vi "TEST - Write INI Cluster.vi"(8 "error in (no error)":errorcluster) -> (0 "error out":errorcluster, 2 "Passed":bool)   [LabVIEW 2009]
uses:
  <vilib>/Utility/config.llb/NI_LVConfig.lvlib
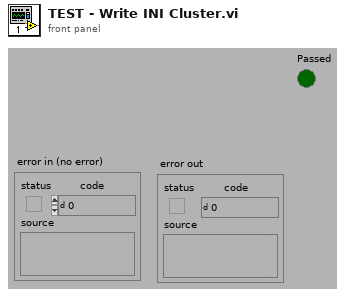
[diagram p1: front panel]
types:
  T1 = cluster{"Section 1":cluster{"Float":dbl, "Integer":i32}, "Section 2":cluster{"Boolean":bool, "String":string}}
  T2 = typedef "NI_LVConfig.lvlib/Config Data RefNum.ctl" = refnum<k1>
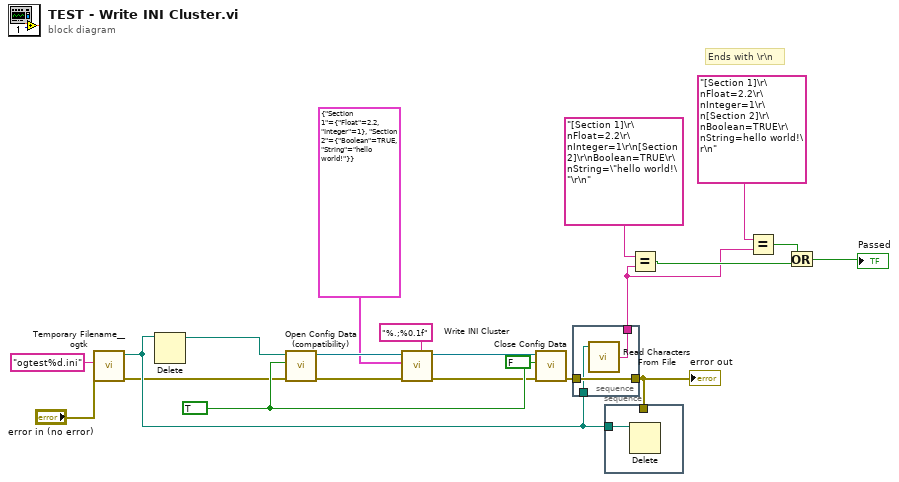
[diagram p0: block diagram]
diagram:
  (unwired) FALSE ("write configuration file? (T)")
  w19 = TRUE ("create file if necessary? (T)")
  # "Ends with \\r\\n"
  n1 = call <userlib>:"Temporary Filename__ogtk.vi"("error in (no error)"="error in (no error)", "pattern (lvtemp%d.tmp)"="ogtest%d.ini") -> ("error out"=w7:errorcluster, "file in tmp dir"=w8:path)  [unwired: 4 in]
  n2 = Delete(path (use dialog)=w8) -> (deleted path=w17:path)  [unwired: 4 in, 2 out]
  n3 = call <vilib>:"Open Config Data (compatibility).vi"("error in (no error)"=w7, "create file if necessary (T)"=w19, "configuration file path"=w17) -> ("error out"=w15:errorcluster, "refnum"=w16:T2)  [unwired: 6 in, 1 out]
  n4 = call "Write INI Cluster.vi"("float number format (optional)"="%.;%0.1f", "error in (no error)"=w15, "INI Fomatted Cluster"=T1 {"Section 1"={"Float"=2.2, "Integer"=1}, "Section 2"={"Boolean"=TRUE, "String"="hello world!"}}, "refnum"=w16) -> ("error out"=w18:errorcluster, "dup refnum"=w20:T2)  [unwired: 6 in]
  n5 = call <vilib>:"Close Config Data.vi"("error in (no error)"=w18, "write file if changed (T)"=w19, "refnum"=w20) -> ("error out"=w13:errorcluster)  [unwired: 7 in, 1 out]
  n6 = stacked-sequence {
    tunnel: w13 -> [w23]
    tunnel: [w23] -> w12
    tunnel: w8 -> [w22]
    tunnel: [w21] -> w2
    frame #0 {
      n7 = call <vilib>:"Read Characters From File.vi"("file path (dialog if empty)"=w22) -> ("character string"=w21:string)  [unwired: 5 in, 3 out]
    }
  }
  "error out" <- w12
  n8 = stacked-sequence {
    tunnel: w8 -> [w24]
    tunnel: w12 -> [_]
    frame #0 {
      n9 = Delete(path (use dialog)=w24) -> ()  [unwired: 4 in, 3 out]
    }
  }
  n10 = Equal?(x="[Section 1]\r\nFloat=2.2\r\nInteger=1\r\n[Section 2]\r\nBoolean=TRUE\r\nString=\"hello world!\"\r\n" ("character string"), y=w2) -> (x = y?=w4:bool)
  n11 = Equal?(x="[Section 1]\r\nFloat=2.2\r\nInteger=1\r\n[Section 2]\r\nBoolean=TRUE\r\nString=hello world!\r\n" ("character string"), y=w2) -> (x = y?=w5:bool)
  n12 = Or(x=w5, y=w4) -> (x .or. y?=→"Passed":bool)
